vi "Save Practice.vi"() -> ()   [LabVIEW 2018]
uses:
  <vilib>/Utility/xml.llb/Write to XML File(string).vi
  <vilib>/Utility/xml.llb/Read From XML File(array).vi
panel:
  out "value":i32[](array[numeric])
  out "appended path":path
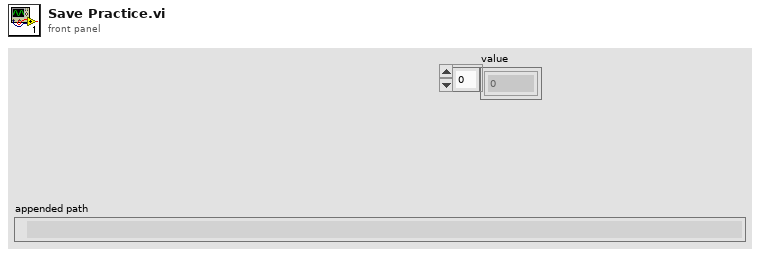
[diagram p1: front panel]
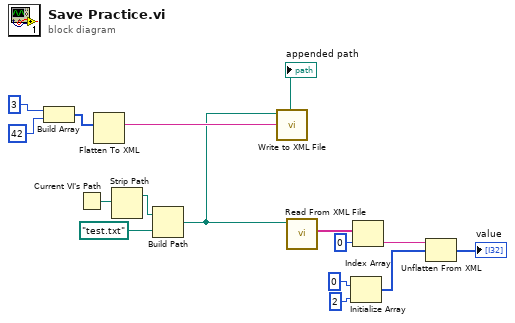
[diagram p0: block diagram]
diagram:
  n1 = Build Array(3, 42) -> (w5:i32[])
  n2 = Current VI's Path() -> (path=w10:path)
  n3 = Flatten To XML(anything=w5) -> (xml string=w15:string)
  n4 = Strip Path(path=w10) -> (stripped path=w11:path)  [unwired: 1 out]
  n5 = Build Path(base path=w11, name or relative path=path "test.txt" ("XML File Path")) -> (appended path=w9:path)
  "appended path" <- w9
  n6 = call-poly <vilib>:"Write to XML File.vi"("XML Input"=w15, "XML File Path"=w9) -> ()  [unwired: 7 in, 3 out]
  n7 = call-poly <vilib>:"Read From XML File.vi"("XML File Path"=w9) -> ("XML Elements"=w8:string[])  [unwired: 8 in, 2 out]
  n8 = Initialize Array(0, 2 ("dimension size")) -> (w2:i32[])
  n9 = Index Array(array=w8, index=0) -> (element=w6:string)
  n10 = Unflatten From XML(xml string=w6, type=w2) -> (value=→"value":i32[])  [unwired: 1 in, 1 out]
